vi "FFTunwrappedResult.vi"(6 "fft cluster acquisition":T2, 9 "sequence NbX NbZ":dbl[][](array[numeric]), 10 "output cluster":T1, 11 "result array out":dbl[][](array[numeric])) -> (1 "image":dbl[][](array[numeric]), 3 "modules FFT":dbl[][](array[numeric]))   [LabVIEW 2018]
uses:
  <vilib>/Analysis/2dsp.llb/2D Inverse Complex FFT.vi
  General Libraries/myFFT.lvlib
  <vilib>/Analysis/NI_AALPro.lvlib
panel:
  out "Array":cdb[][](array[numeric])
  out "Intensity Graph":dbl[][](graph)
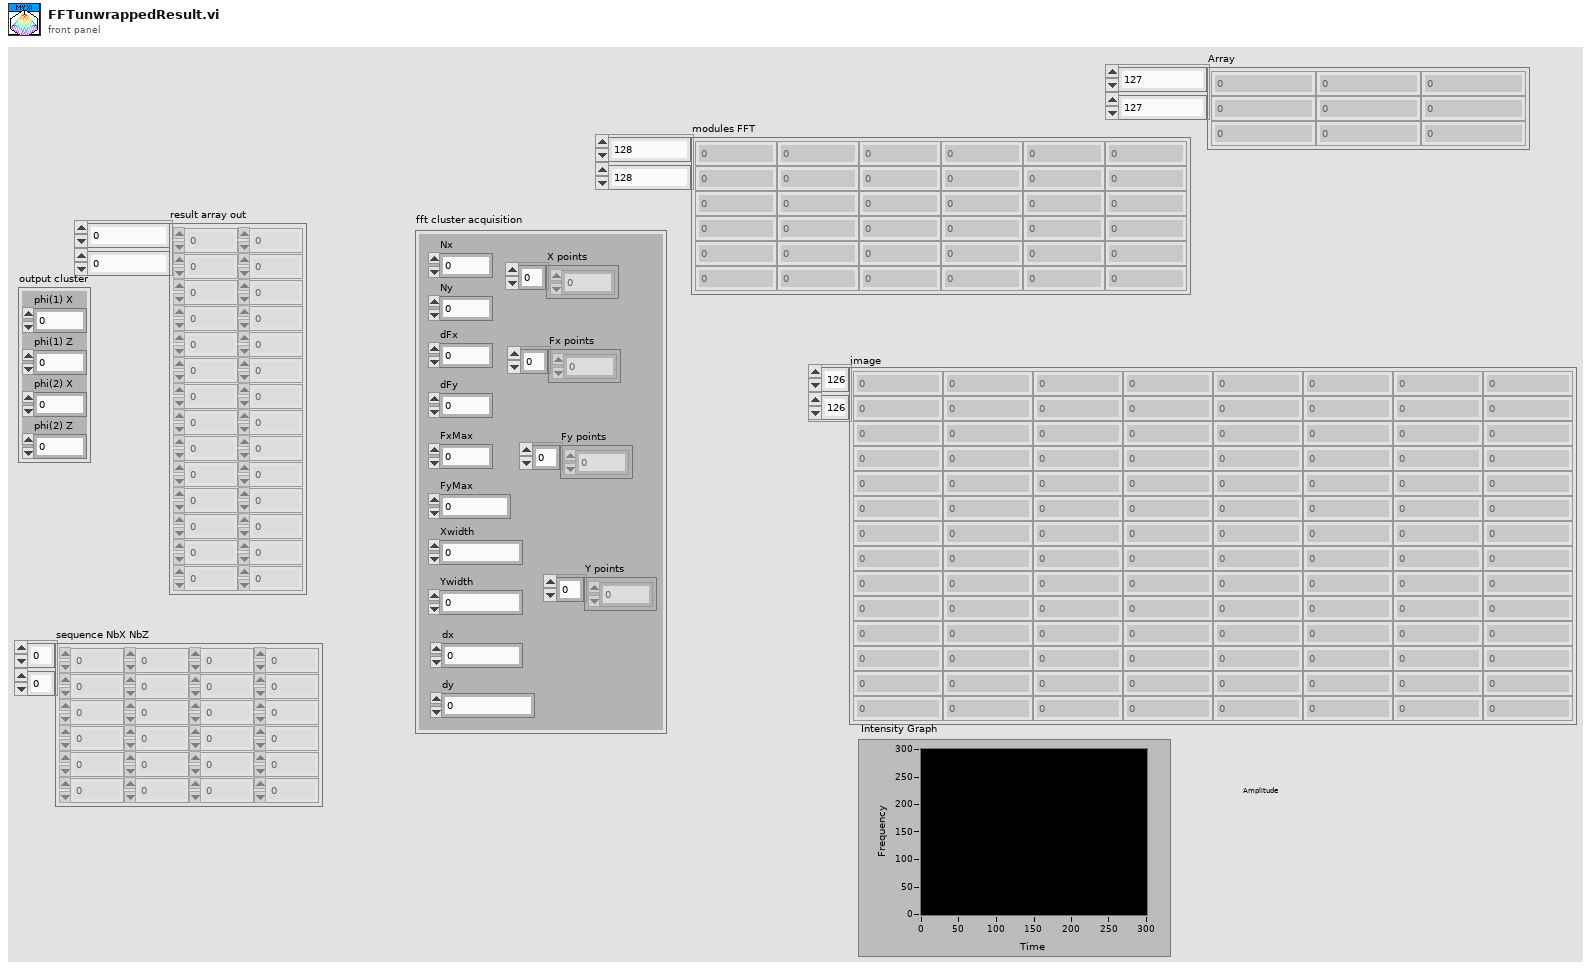
[diagram p1: front panel]
types:
  T1 = cluster{"phi(1) X":dbl, "phi(1) Z":dbl, "phi(2) X":dbl, "phi(2) Z":dbl}
  T2 = cluster{"dFx":dbl, "dFy":dbl, "Nx":i32, "Ny":i32, "FxMax":dbl, "FyMax":dbl, "Xwidth":dbl, "Ywidth":dbl, "dx":dbl, "dy":dbl, "Fx points":dbl[], "X points":dbl[], "Y points":dbl[], "Fy points":dbl[]}
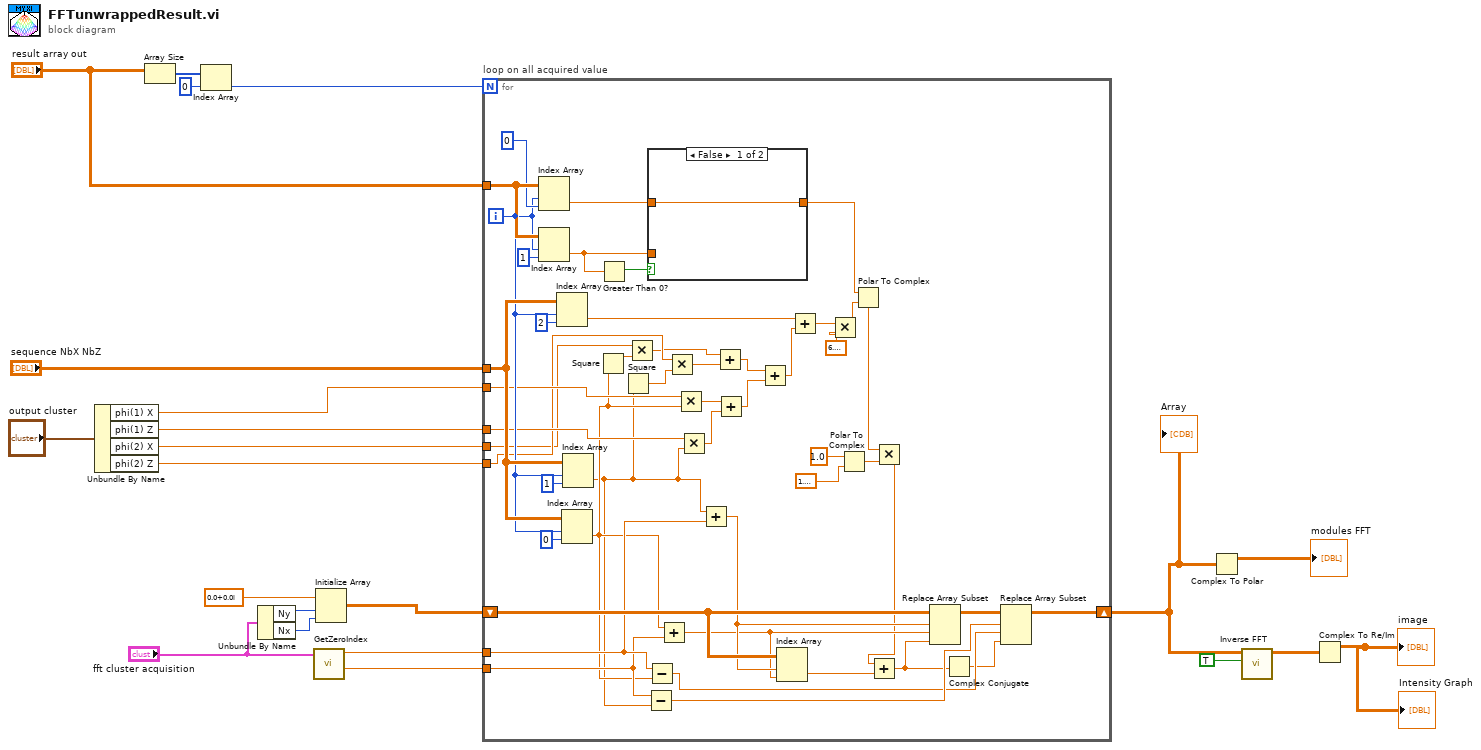
[diagram p0: block diagram]
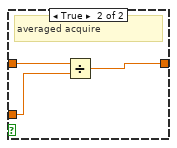
[diagram p2: hidden frame]
diagram:
  n1 = Unbundle By Name("output cluster") -> ("phi(1) X"=w6:dbl, "phi(1) Z"=w5:dbl, "phi(2) X"=w4:dbl, "phi(2) Z"=w3:dbl)
  n2 = Array Size(array="result array out") -> (size(s)=w22:i32[])
  n3 = Index Array(array=w22, index=0) -> (element=w20:i32)
  n4 = Unbundle By Name("fft cluster acquisition") -> ("Ny"=w14:i32, "Nx"=w13:i32)
  n5 = call "GetZeroIndex.vi"("fft cluster"="fft cluster acquisition") -> ("Nx/2+1"=w16:dbl, "Ny/2+1"=w17:dbl)  [unwired: 9 in]
  n6 = Initialize Array(cdb 0.0+0.0i ("element"), w14, w13) -> (w12:cdb[][])
  n7 = for "loop on all acquired value" {
    N: w20 -> [_]
    tunnel: "sequence NbX NbZ" -> [w60]
    tunnel: "result array out" -> [w70]
    tunnel: w17 -> [w51]
    tunnel: w16 -> [w50]
    shift-right: [w47] -> w8
    shift-left: w12 -> [w56]
    tunnel: w6 -> [w40]
    tunnel: w5 -> [w39]
    tunnel: w4 -> [w34]
    tunnel: w3 -> [w35]
    i -> [w59]
    n8 = Index Array(array=w70, index (row)=w59, index (col)=0 ("disabled index (col)")) -> (element=w68:dbl)
    n9 = Index Array(array=w70, index (row)=w59, index (col)=1 ("disabled index (col)")) -> (element=w66:dbl)
    n10 = Index Array(array=w60, index (row)=w59, index (col)=2 ("disabled index (col)")) -> (element=w44:dbl)
    n11 = Index Array(array=w60, index (row)=w59, index (col)=0 ("disabled index (col)")) -> (element=w31:dbl)
    n12 = Index Array(array=w60, index (row)=w59, index (col)=1 ("disabled index (col)")) -> (element=w29:dbl)
    n13 = Square(x=w31) -> (x^2=w30:dbl)
    n14 = Greater Than 0?(x=w66) -> (x > 0?=w67:bool)
    n15 = Square(x=w29) -> (x^2=w28:dbl)
    n16 = Multiply(x=w34, y=w30) -> (x*y=w33:dbl)
    n17 = Subtract(x=w50, y=w29) -> (x-y=w49:dbl)
    n18 = Subtract(x=w51, y=w31) -> (x-y=w48:dbl)
    n19 = case shown="False" w67 {
      tunnel: w68 -> [w71 w74]
      tunnel: w66 -> [_ w73]
      tunnel: [w71 w72] -> w62
      frame False {
      }
      frame True {
        # "averaged acquire"
        n20 = Divide(x=w74, y=w73) -> (x/y=w72:dbl)
      }
    }
    n21 = Add(x=w31, y=w50) -> (x+y=w54:dbl)
    n22 = Multiply(x=w35, y=w28) -> (x*y=w32:dbl)
    n23 = Multiply(x=w40, y=w31) -> (x*y=w42:dbl)
    n24 = Multiply(x=w39, y=w29) -> (x*y=w41:dbl)
    n25 = Add(x=w29, y=w51) -> (x+y=w55:dbl)
    n26 = Add(x=w33, y=w32) -> (x+y=w38:dbl)
    n27 = Add(x=w42, y=w41) -> (x+y=w37:dbl)
    n28 = Add(x=w38, y=w37) -> (x+y=w36:dbl)
    n29 = Index Array(array=w56, index (row)=w55, index (col)=w54) -> (element=w53:cdb)
    n30 = Add(x=w44, y=w36) -> (x+y=w43:dbl)
    n31 = Multiply(x=w43, y=6.283185307179586) -> (x*y=w61:dbl)
    n32 = Polar To Complex(1:1.5707963267948966, 2:1.0 ("r")) -> (0:w25:cdb)
    n33 = Polar To Complex(1:w61, 2:w62) -> (0:w27:cdb)
    n34 = Multiply(x=w27, y=w25) -> (x*y=w26:cdb)
    n35 = Add(x=w26, y=w53) -> (x+y=w46:cdb)
    n36 = Replace Array Subset(array=w56, new element=w46, index (row)=w55, index (col)=w54) -> (w52:cdb[][])
    n37 = Complex Conjugate(1:w46) -> (0:w45:cdb)
    n38 = Replace Array Subset(array=w52, new element=w45, index (row)=w49, index (col)=w48) -> (w47:cdb[][])
  }
  "Array" <- w8
  n39 = Complex To Polar(r * e^(i*theta)=w8) -> (r=→"modules FFT":dbl[][])  [unwired: 1 out]
  n40 = call-poly <vilib>:"Inverse FFT.vi"("shift?"=TRUE, "FFT {x}"=w8) -> ("X"=w2:cdb[][])  [unwired: 8 in, 1 out]
  n41 = Complex To Re/Im(x + iy=w2) -> (x=→"image" →"Intensity Graph":dbl[][])  [unwired: 1 out]
